vi "Hex to Colorbox.vi"() -> ()   [LabVIEW 2019]
panel:
  out "Array 2":u32[](array[colorbox])
  out "Array":string[](array[string])
  out "array":string[](array[string])
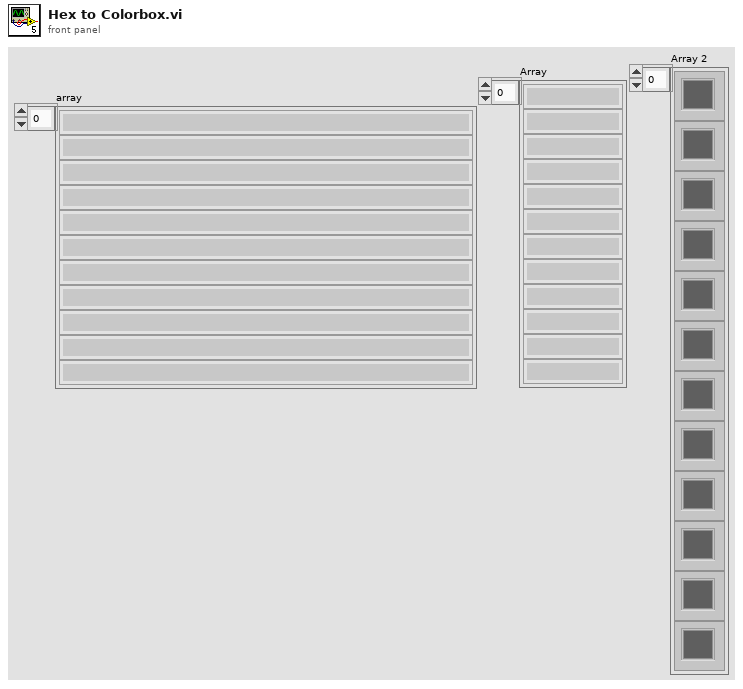
[diagram p1: front panel]
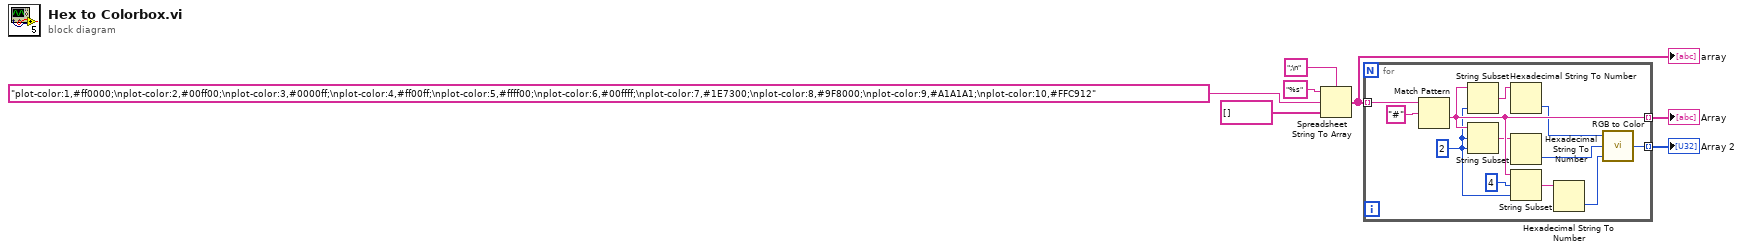
[diagram p0: block diagram]
diagram:
  n1 = Spreadsheet String To Array(delimiter (Tab)=";\n", format string="%s", spreadsheet string="plot-color:1,#ff0000;\nplot-color:2,#00ff00;\nplot-color:3,#0000ff;\nplot-color:4,#ff00ff;\nplot-color:5,#ffff00;\nplot-color:6,#00ffff;\nplot-color:7,#1E7300;\nplot-color:8,#9F8000;\nplot-color:9,#A1A1A1;\nplot-color:10,#FFC912", array type (2D Dbl)=string[] [] ("format string")) -> (array=w3:string[])
  "array" <- w3
  n2 = for {
    tunnel: w3 -> [w19] mode=indexing
    tunnel: [w17] -> w2 mode=indexing
    tunnel: [w8] -> w1 mode=indexing
    w16 = 2 ("length (rest)")
    n3 = Match Pattern(string=w19, regular expression="#") -> (after substring=w17:string)  [unwired: 1 in, 3 out]
    n4 = String Subset(string=w17, length (rest)=w16) -> (substring=w14:string)  [unwired: 1 in]
    n5 = String Subset(string=w17, offset (0)=w16, length (rest)=w16) -> (substring=w12:string)
    n6 = Hexadecimal String To Number(string=w14) -> (number=w13:u32)  [unwired: 2 in, 1 out]
    n7 = Hexadecimal String To Number(string=w12) -> (number=w11:u32)  [unwired: 2 in, 1 out]
    n8 = String Subset(string=w17, offset (0)=4, length (rest)=w16) -> (substring=w10:string)
    n9 = Hexadecimal String To Number(string=w10) -> (number=w9:u32)  [unwired: 2 in, 1 out]
    n10 = call <vilib>:"RGB to Color.vi"("B"=w9, "G"=w11, "R"=w13) -> ("Color"=w8:u32)
  }
  "Array" <- w2
  "Array 2" <- w1
